vi "HW_Poll_Tracker_2.0.4+.vi"(8 "error in":errorcluster, 11 "VISA resource name in":refnum<visa-resource-name>="ASRL3::INSTR") -> (0 "error out":errorcluster, 1 "Read buffer":string, 2 "Parameters output":T1, 3 "VISA resource name out":refnum<visa-resource-name>, 4 "Sync mode status":string, 5 "Sensor board size":string)   [LabVIEW 2018]
panel:
  out "Sync mode index":i32
  out "Sensor board index":i32
  out "Sensors response":string
  out "Port data status":i32
  out "Port data status index":i32
  out "FPS status":i32
  out "Poll records":u32
  out "FPS target index":i32
  out "Matrix mode status":string
  out "Matrix mode index":i32
  out "Coordinate mode status":string
  out "Coordinate mode index":i32
  out "Binary mode status":string
  out "Binary mode index":i32
  out "Array of tokens":string[](array[string])
  out "token index":i32
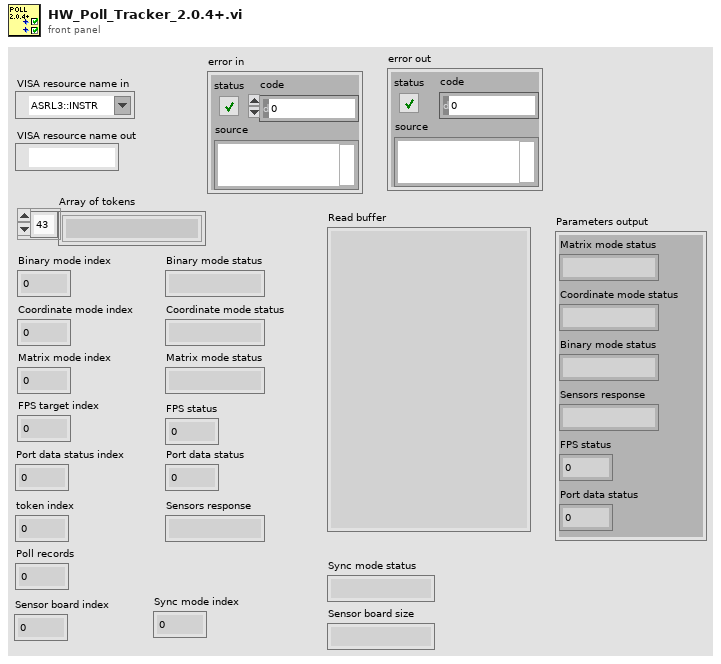
[diagram p1: front panel]
types:
  T1 = cluster{"Matrix mode status":string, "Coordinate mode status":string, "Binary mode status":string, "Sensors response":string, "FPS status":i32, "Port data status":i32}
  T2 = cluster{"token string":string, "token string":string, "token string":string, "trimmed string":string, i32, i32}
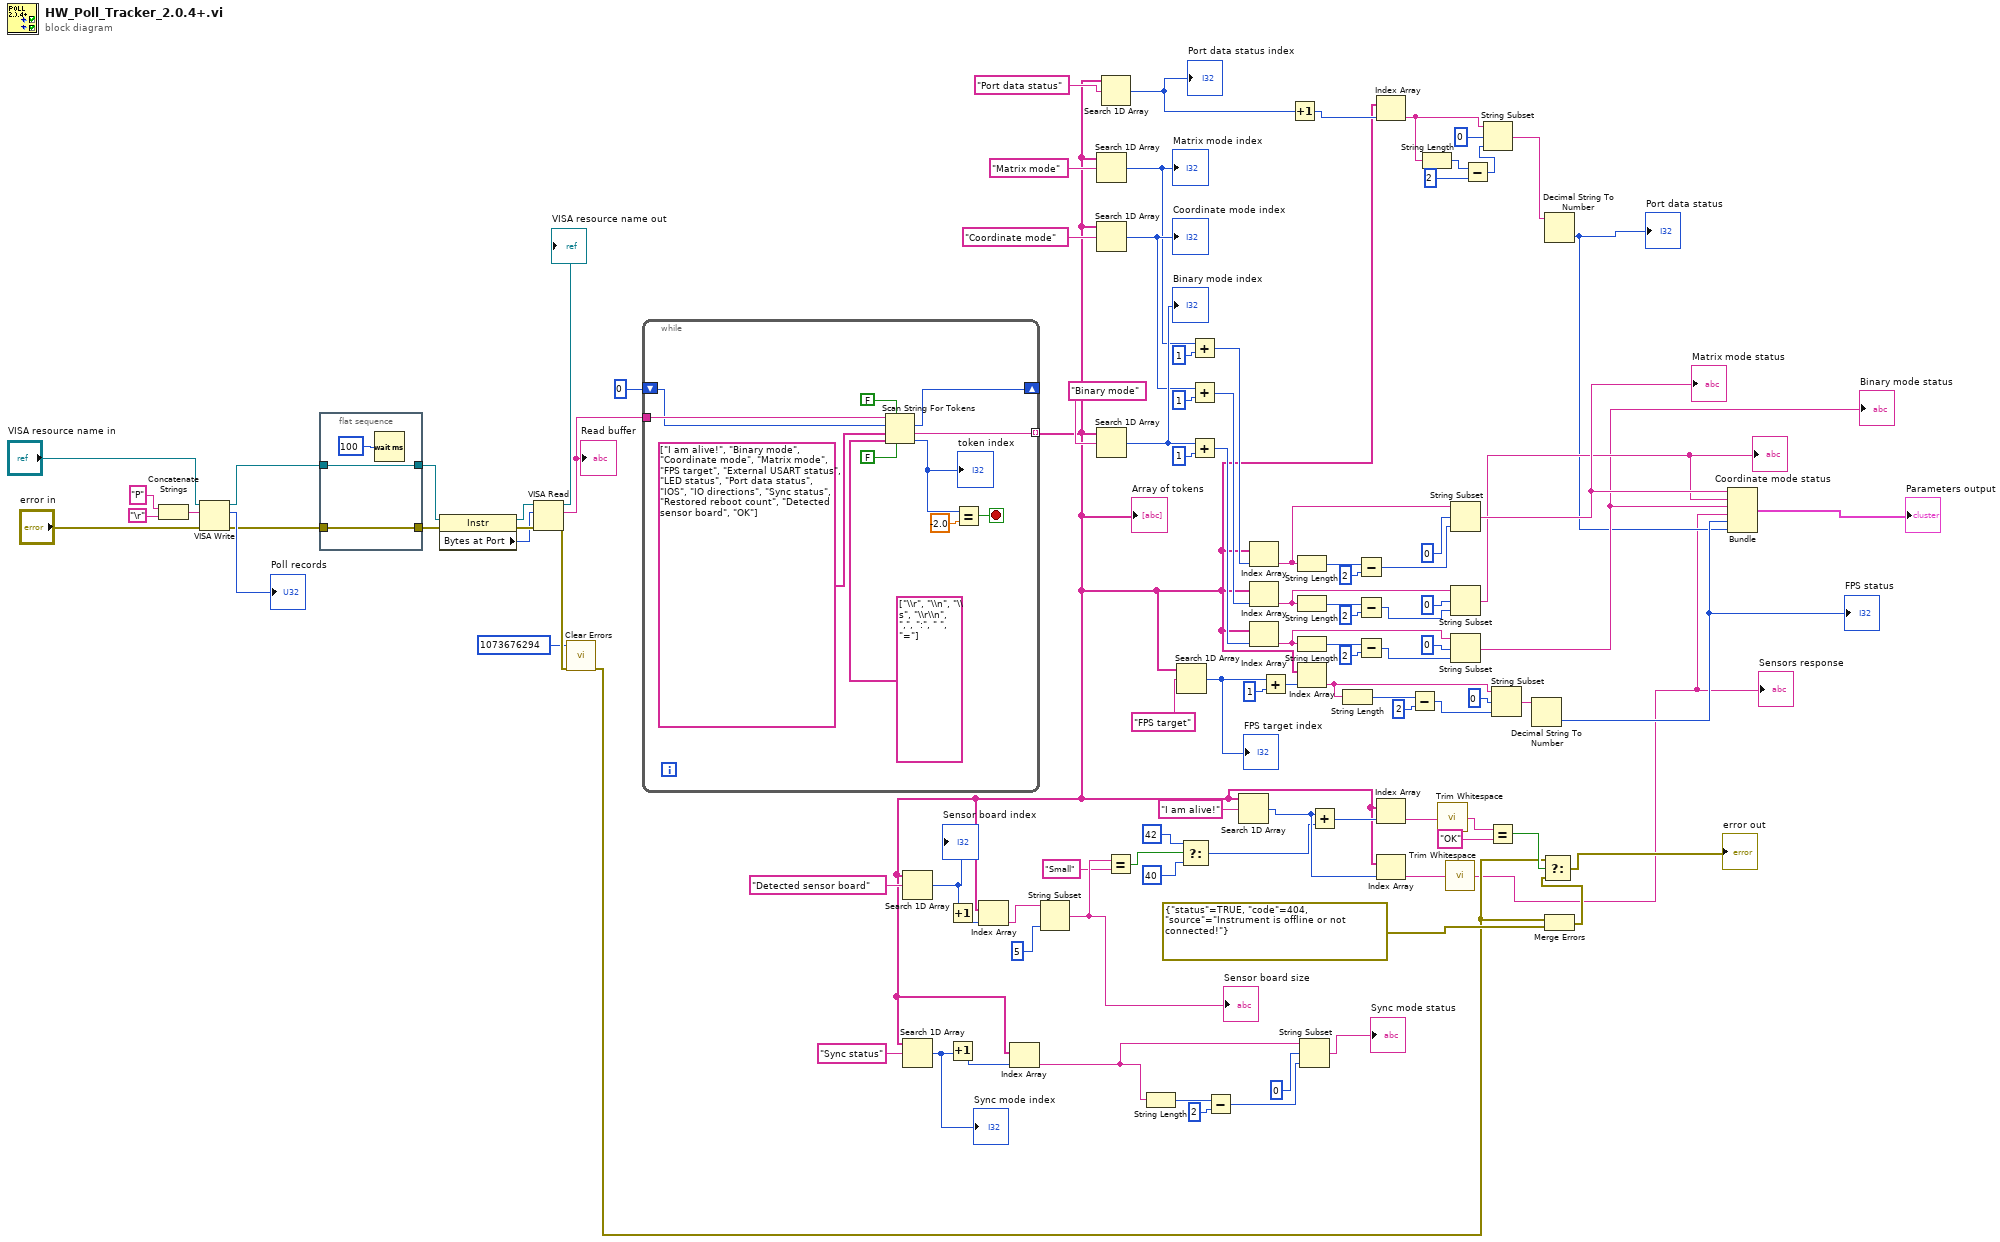
[diagram p0: block diagram]
diagram:
  n1 = Concatenate Strings("P" ("write buffer"), "\r") -> (w102:string)
  n2 = VISA Write(VISA resource name="VISA resource name in", write buffer=w102, error in (no error)="error in") -> (VISA resource name out=w77:refnum<visa-resource-name>, return count=→"Poll records":u32, error out=w75:errorcluster)
  n3 = flat-sequence {
    tunnel: [w106] -> w78
    tunnel: w77 -> [w106]
    tunnel: [w105] -> w76
    tunnel: w75 -> [w105]
    frame #0 {
      n4 = Wait (ms)(milliseconds to wait=u32 100) -> ()  [unwired: 1 out]
    }
  }
  n5 = property class="Instr"(reference=w78, error in=w76) -> (reference out=w100:refnum<visa-resource-name>, error out=w99:errorcluster, "Bytes at Port"=w98:u32)
  n6 = VISA Read(VISA resource name=w100, byte count=w98, error in (no error)=w99) -> (VISA resource name out=→"VISA resource name out":refnum<visa-resource-name>, read buffer=w97:string, error out=w35:errorcluster)  [unwired: 1 out]
  "Read buffer" <- w97
  n7 = call <vilib>:"Clear Errors.vi"("error in (no error)"=w35, "specific error code to clear (0: all)"=1073676294) -> ("error out"=w34:errorcluster)  [unwired: 4 in, 1 out]
  n8 = while {
    tunnel: w97 -> [w118]
    tunnel: [w110] -> w18 mode=indexing
    shift-right: [w109] -> _
    shift-left: 0 ("offset past token") -> [w108]
    stop <- w116 stop-if-true
    n9 = Scan String For Tokens(4:FALSE ("use cached delim/oper data? (F)"), 5:FALSE ("allow empty tokens? (F)"), 6:string[] ["\\r", "\\n", "\\s", "\\r\\n", ",", ":", " ", "="] ("delimiters"), 7:string[] ["I am alive!", "Binary mode", "Coordinate mode", "Matrix mode", "FPS target", "External USART status", "LED status", "Port data status", "IOS", "IO directions", "Sync status", "Restored reboot count", "Detected sensor board", "OK"] ("Tokens"), 8:w108, 9:w118) -> (0:w114:i32, 1:w110:string, 2:w109:i32)  [unwired: 1 out]
    "token index" <- w114
    n10 = Equal?(x=w114, y=-2.0) -> (x = y?=w116:bool)
  }
  "Array of tokens" <- w18
  n11 = Search 1D Array(1D array=w18, element="Detected sensor board") -> (index of element=w24:i32)  [unwired: 1 in]
  "Sensor board index" <- w24
  n12 = Search 1D Array(1D array=w18, element="Sync status") -> (index of element=w11:i32)  [unwired: 1 in]
  "Sync mode index" <- w11
  n13 = Increment(x=w24) -> (x+1=w23:i32)
  n14 = Increment(x=w11) -> (x+1=w19:i32)
  n15 = Index Array(array=w18, index=w23) -> (element=w22:string)
  n16 = Index Array(array=w18, index=w19) -> (element=w12:string)
  n17 = String Subset(string=w22, length (rest)=5 ("length (rest)")) -> (substring=w7:string)  [unwired: 1 in]
  "Sensor board size" <- w7
  n18 = Search 1D Array(1D array=w18, element="Matrix mode") -> (index of element=w86:i32)  [unwired: 1 in]
  "Matrix mode index" <- w86
  n19 = Search 1D Array(1D array=w18, element="Coordinate mode") -> (index of element=w90:i32)  [unwired: 1 in]
  "Coordinate mode index" <- w90
  n20 = Search 1D Array(1D array=w18, element="Binary mode") -> (index of element=w94:i32)  [unwired: 1 in]
  "Binary mode index" <- w94
  n21 = Search 1D Array(1D array=w18, element="Port data status") -> (index of element=w51:i32)  [unwired: 1 in]
  "Port data status index" <- w51
  n22 = Equal?(x=w7, y="Small") -> (x = y?=w5:bool)
  n23 = String Length(string=w12) -> (length=w15:i32)
  n24 = Search 1D Array(1D array=w18, element="FPS target") -> (index of element=w82:i32)  [unwired: 1 in]
  "FPS target index" <- w82
  n25 = Select(t=42, s=w5, f=40 ("y")) -> (s? t:f=w3:i32)
  n26 = Add(x=w86, y=1) -> (x+y=w87:i32)
  n27 = Add(x=w90, y=1) -> (x+y=w91:i32)
  n28 = Add(x=w94, y=1) -> (x+y=w95:i32)
  n29 = Subtract(x=w15, y=2) -> (x-y=w17:i32)
  n30 = Search 1D Array(1D array=w18, element="I am alive!") -> (index of element=w10:i32)  [unwired: 1 in]
  n31 = Index Array(array=w18, index=w87) -> (element=w55:string)
  n32 = Index Array(array=w18, index=w91) -> (element=w53:string)
  n33 = Index Array(array=w18, index=w95) -> (element=w72:string)
  n34 = Add(x=w82, y=1) -> (x+y=w83:i32)
  n35 = Increment(x=w51) -> (x+1=w50:i32)
  n36 = String Length(string=w55) -> (length=w67:i32)
  n37 = String Length(string=w53) -> (length=w58:i32)
  n38 = String Length(string=w72) -> (length=w71:i32)
  n39 = Index Array(array=w18, index=w83) -> (element=w54:string)
  n40 = String Subset(string=w12, offset (0)=0, length (rest)=w17) -> (substring=→"Sync mode status":string)
  n41 = Add(x=w10, y=w3) -> (x+y=w32:i32)
  n42 = String Length(string=w54) -> (length=w63:i32)
  n43 = Subtract(x=w67, y=2) -> (x-y=w65:i32)
  n44 = Subtract(x=w58, y=2) -> (x-y=w56:i32)
  n45 = Subtract(x=w71, y=2) -> (x-y=w69:i32)
  n46 = Index Array(array=w18, index=w50) -> (element=w49:string)
  n47 = Index Array(array=w18, index=w32) -> (element=w42:string)
  n48 = Index Array(array=w18, index=w10) -> (element=w9:string)
  n49 = Subtract(x=w63, y=2) -> (x-y=w61:i32)
  n50 = String Length(string=w49) -> (length=w48:i32)
  n51 = call <vilib>:"Trim Whitespace.vi"("string"=w42) -> ("trimmed string"=w41:string)  [unwired: 1 in]
  n52 = call <vilib>:"Trim Whitespace.vi"("string"=w9) -> ("trimmed string"=w8:string)  [unwired: 1 in]
  "Sensors response" <- w8
  n53 = String Subset(string=w55, offset (0)=0, length (rest)=w65) -> (substring=w31:string)
  "Matrix mode status" <- w31
  n54 = String Subset(string=w53, offset (0)=0, length (rest)=w56) -> (substring=w30:string)
  "Coordinate mode status" <- w30
  n55 = String Subset(string=w72, offset (0)=0, length (rest)=w69) -> (substring=w29:string)
  "Binary mode status" <- w29
  n56 = Subtract(x=w48, y=2) -> (x-y=w46:i32)
  n57 = String Subset(string=w49, offset (0)=0, length (rest)=w46) -> (substring=w44:string)
  n58 = Equal?(x=w41, y="OK") -> (x = y?=w39:bool)
  n59 = String Subset(string=w54, offset (0)=0, length (rest)=w61) -> (substring=w60:string)
  n60 = Decimal String To Number(string=w60) -> (number=w28:i32)  [unwired: 2 in, 1 out]
  "FPS status" <- w28
  n61 = Decimal String To Number(string=w44) -> (number=w27:i32)  [unwired: 2 in, 1 out]
  "Port data status" <- w27
  n62 = Merge Errors(w34, errorcluster {"status"=TRUE, "code"=404, "source"="Instrument is offline or not connected!"} ("error in")) -> (w37:errorcluster)
  n63 = Select(t=w34, s=w39, f=w37) -> (s? t:f=→"error out":errorcluster)
  n64 = Bundle("token string"=w31, "token string"=w30, "token string"=w29, "trimmed string"=w8, w28, w27) -> (→"Parameters output":T2)  [unwired: 1 in]
